vi "Write GroupName.vi"(8 "error in (no error)":errorcluster, 10 "GroupName":string, 11 "VariableGroup in":refnum<class "VariableGroup.lvclass">) -> (0 "error out":errorcluster, 3 "VariableGroup out":refnum<class "VariableGroup.lvclass">)   [LabVIEW 2013, in "VariableGroup.lvclass"]
uses:
  VariableGroup.lvclass
  VariableGroup.lvclass/VariableGroup.ctl
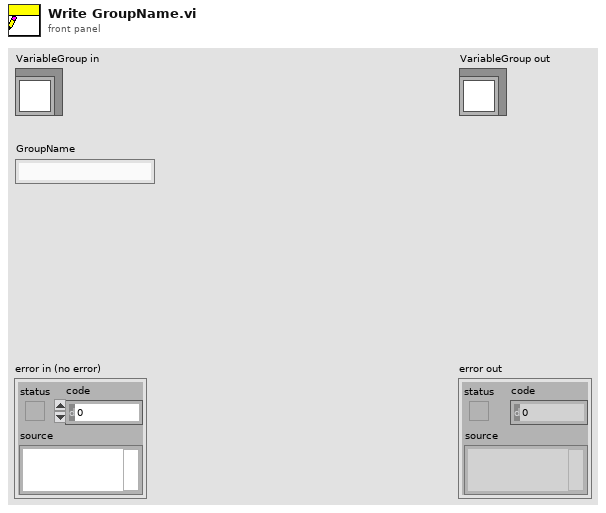
[diagram p1: front panel]
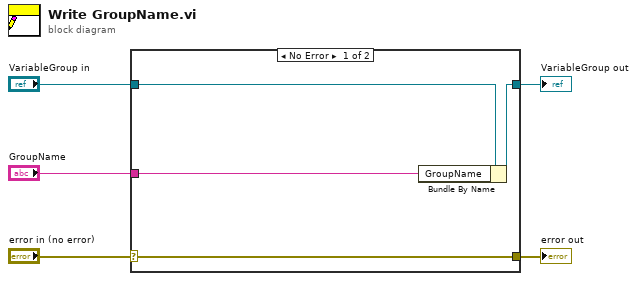
[diagram p0: block diagram]
diagram:
  n1 = case shown="No Error" "error in (no error)" {
    selector: "error in (no error)" -> [w9 w10]
    tunnel: [w9 w10] -> w4
    tunnel: [w7 w11] -> w2
    tunnel: "VariableGroup in" -> [w8 w11]
    tunnel: "GroupName" -> [w6 _]
    frame No Error {
      n2 = Bundle By Name(cluster=w8, "GroupName"=w6) -> (w7:refnum<class "VariableGroup.lvclass">)
    }
    frame Error {
    }
  }
  "error out" <- w4
  "VariableGroup out" <- w2
